vi "tsdiag_can_delete.vi"(8 "错误输入（无错误）":errorcluster, 10 "ADiagModuleIndex":i32, 11 "path":path) -> (0 "错误输出":errorcluster, 2 "Return Type":i32, 3 "path out":path)   [LabVIEW 2014]
doc: "Function Introduction :\nDelete the specified CAN UDS diagnostic service\nCall location :\ninput parameter :\nADiagModulus Index: Save the int pointer of the UDS module, which is used by all diagnostic APIs\nCreate a handle\nReturn value :\n==0: Execution successful\nOther values: Query error code"
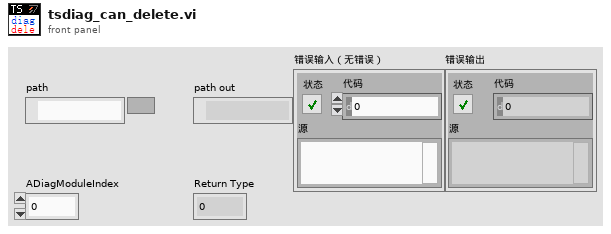
[diagram p1: front panel]
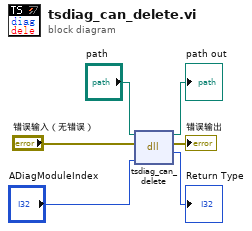
[diagram p0: block diagram]
diagram:
  n1 = dll-call lib="C:/Users/XYY/Desktop/LabView Demo/TSCAN_LB2018_V1.4_20220309/Config/TSMaster.dll" fn="tsdiag_can_delete"(path in="path", error in="错误输入（无错误）", "ADiagModuleIndex"="ADiagModuleIndex") -> (path out=→"path out":path, error out=→"错误输出":errorcluster, "返回类型"=→"Return Type":i32)  [unwired: 2 in]
